vi "1. JKISM vs CSM.vi"() -> ()   [LabVIEW 2017]
uses:
  user.lib/_NEVSTOP/Communicable State Machine(CSM)/AdvanceAPI/CSM - Revert Arguments-Safe String.vi
  user.lib/_NEVSTOP/Communicable State Machine(CSM)/AdvanceAPI/CSM - Make String Arguments Safe.vi
  user.lib/_NEVSTOP/Communicable State Machine(CSM)/AdvanceAPI/CSM - Break Down Multiple States String.vi
  user.lib/_NEVSTOP/Communicable State Machine(CSM)/AdvanceAPI/CSM - Compact Multiple States.vi
  user.lib/_NEVSTOP/Communicable State Machine(CSM)/AdvanceAPI/CSM - Keywords.vi
  user.lib/_NEVSTOP/Communicable State Machine(CSM)/_Shared/Trim Single-line Text.vi
  user.lib/_NEVSTOP/Communicable State Machine(CSM)/Communicable State Machine.lvlib
panel:
  out "State History":string
  in  "Name (\"\" to Use UUID)":string="Event CSM"
  in  "Exit":bool
  # "Demonstrates the framework structures of the JKISM and CSM state machine templates. Both frameworks use string-based message queues to implement the core state machine."
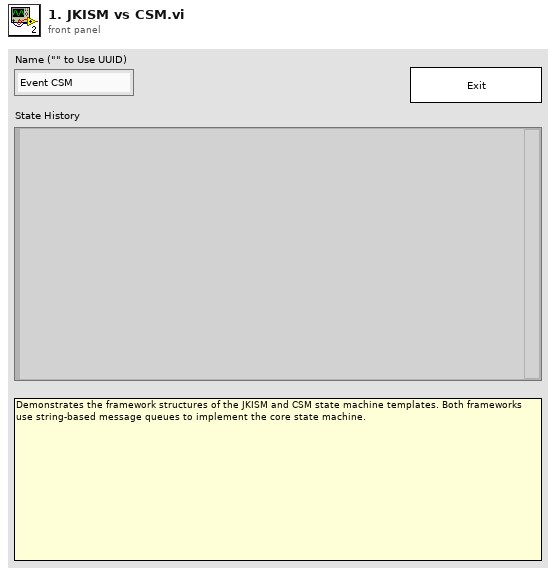
[diagram p1: front panel]
types:
  T1 = enum32{"Invalid", "Standard", "Closed", "Hidden", "Minimized", "Maximized"}
  T2 = enum32{"invalid app kind", "Development System", "Run Time System", "Student Edition", "Embedded LabVIEW", "Evaluation", "Custom"}
  T3 = cluster{"Core":cluster{"Current VI Reference":refnum<vi>, "Close Panel on Exit?":bool}, "Your Boolean data":bool, "Your string data":string}
  T4 = cluster{"Current VI Reference":refnum<vi>, "Close Panel on Exit?":bool}
  T5 = typedef "Communicable State Machine.lvlib/_CSM_Response Source Message.ctl" = cluster{"‘State":string, "’Arguments":string, "’Error":errorcluster}
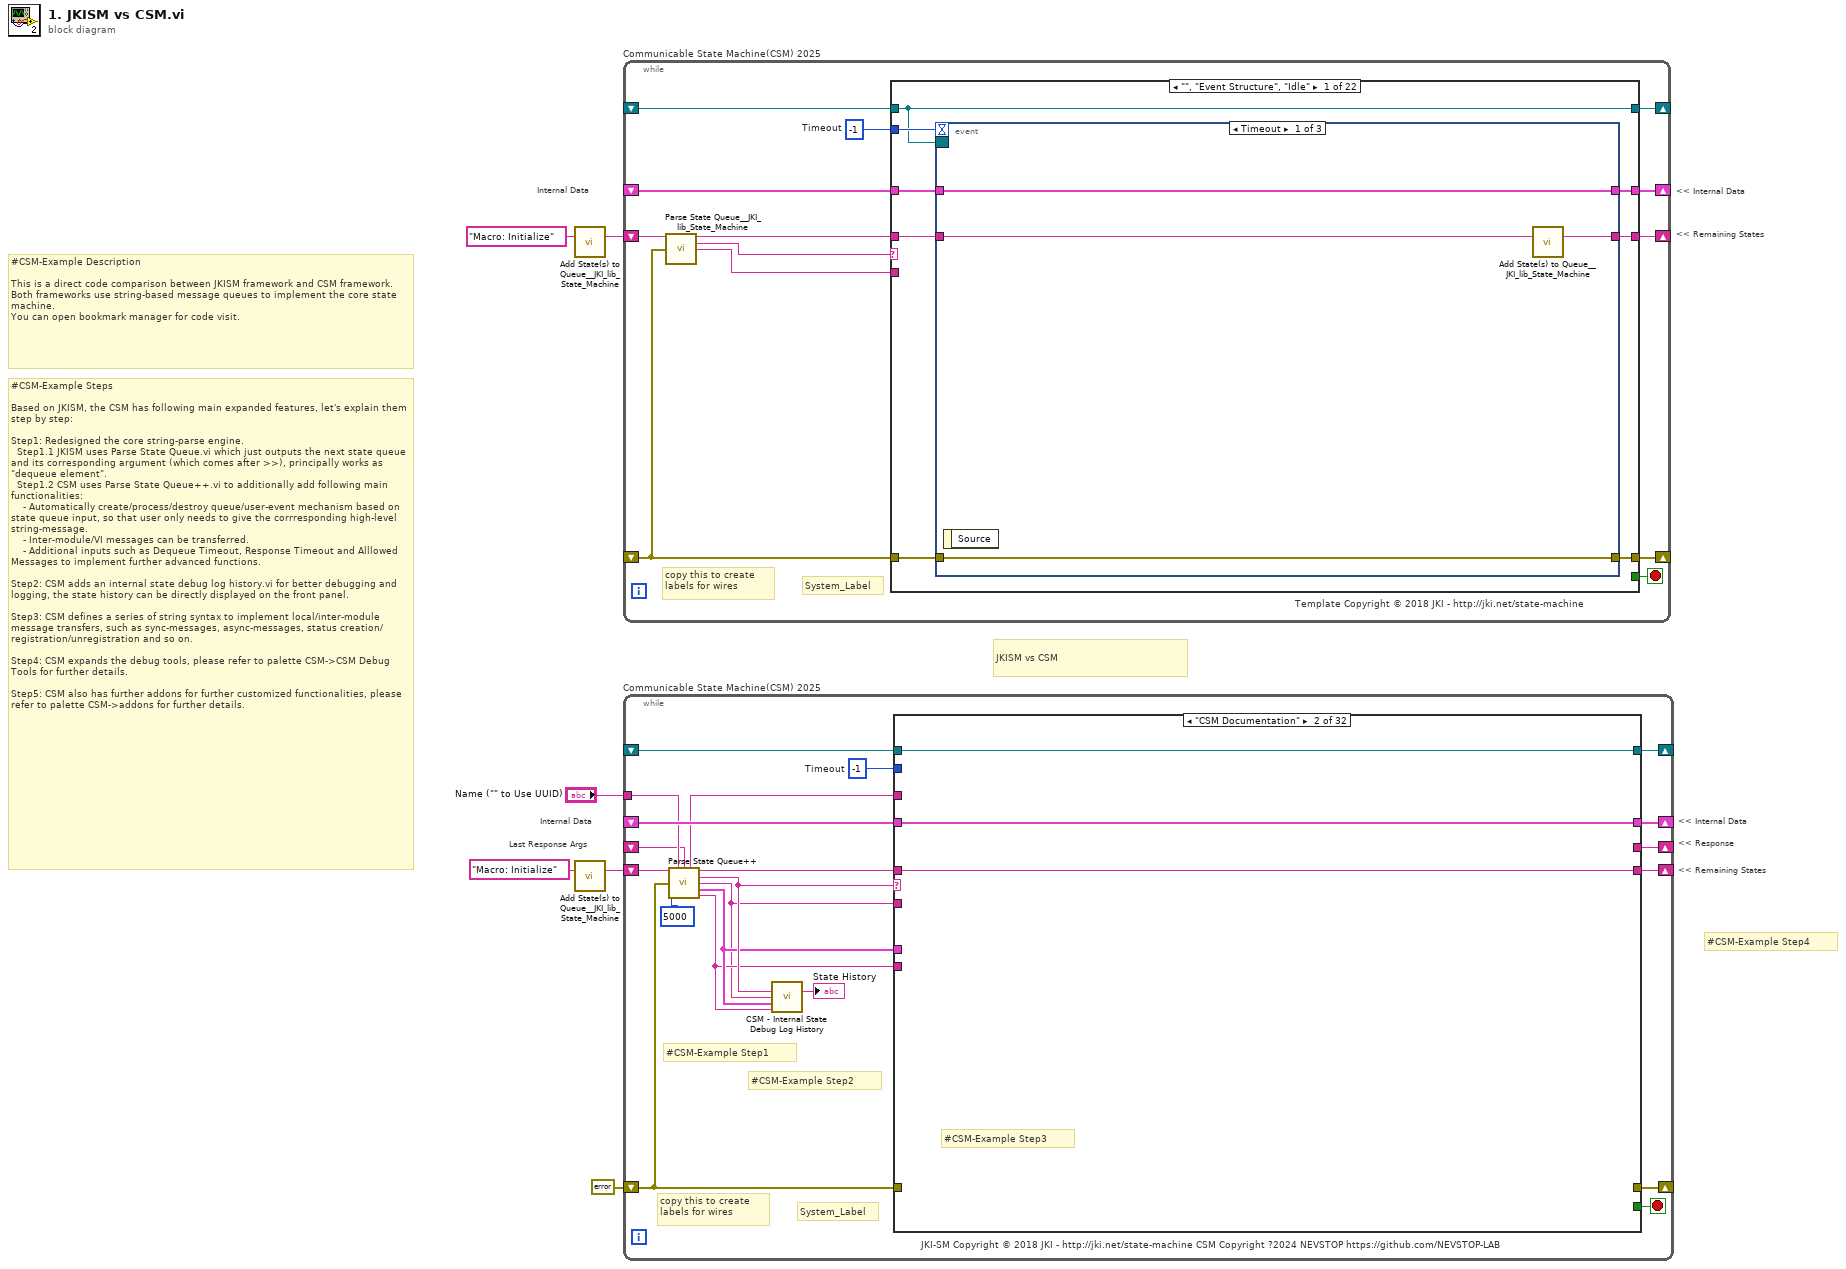
[diagram p0: block diagram]
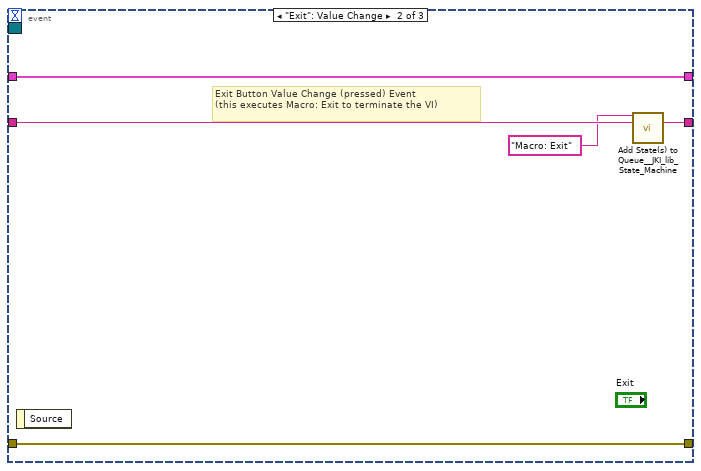
[diagram p2: hidden frame]
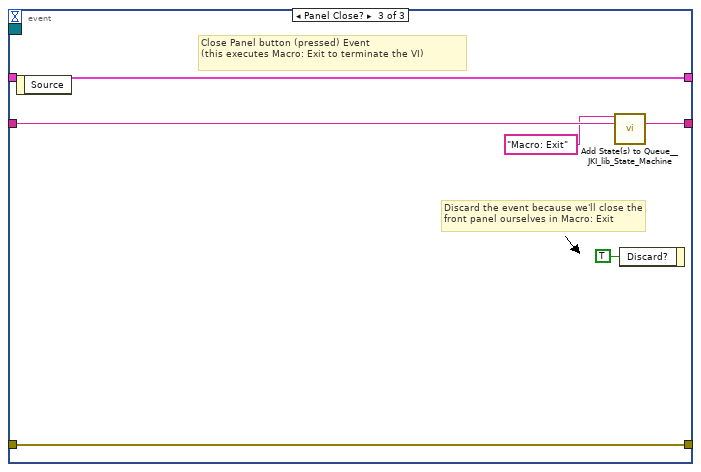
[diagram p3: hidden frame]
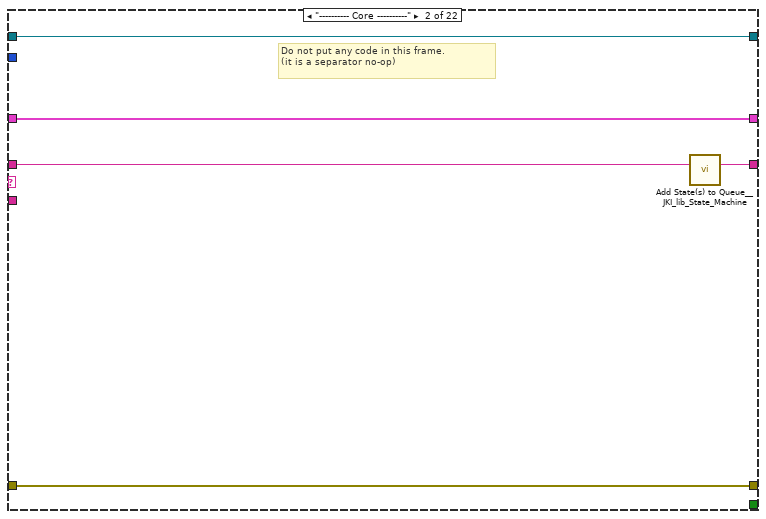
[diagram p4: hidden frame]
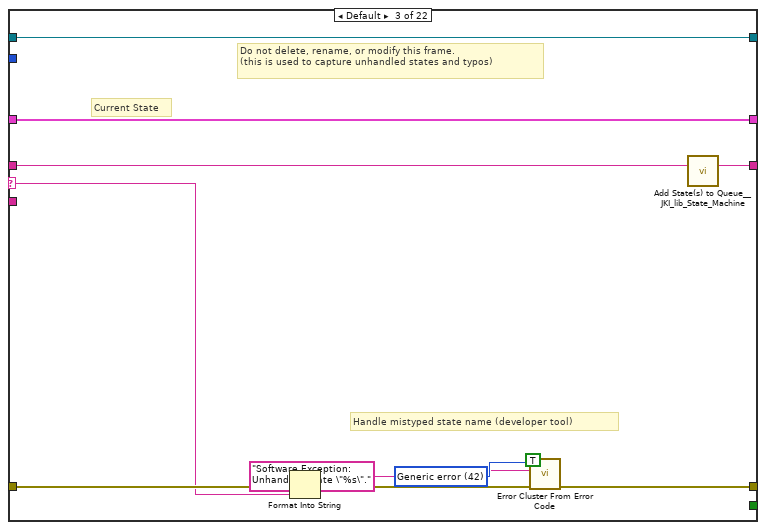
[diagram p5: hidden frame]
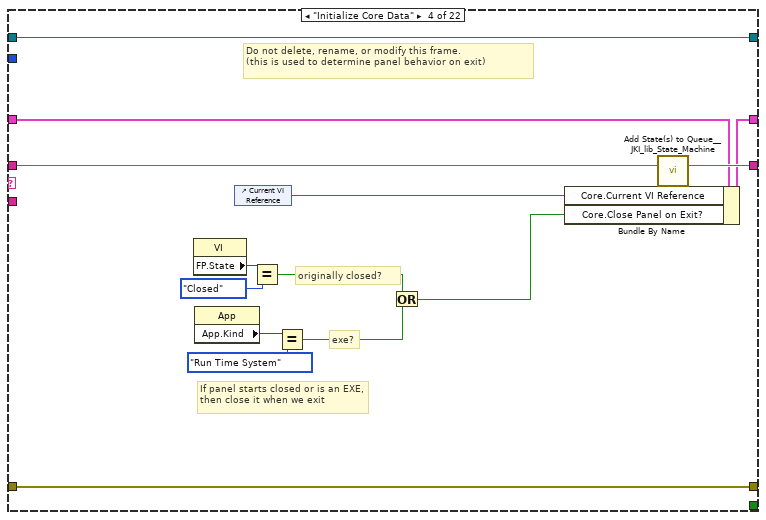
[diagram p6: hidden frame]
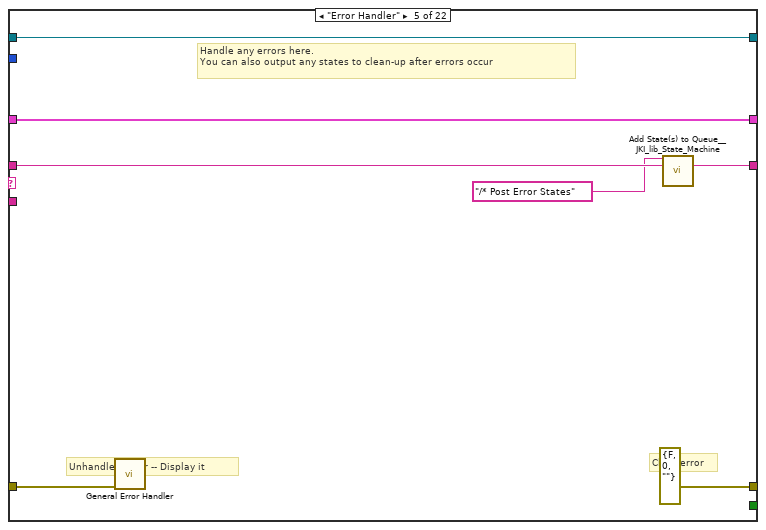
[diagram p7: hidden frame]
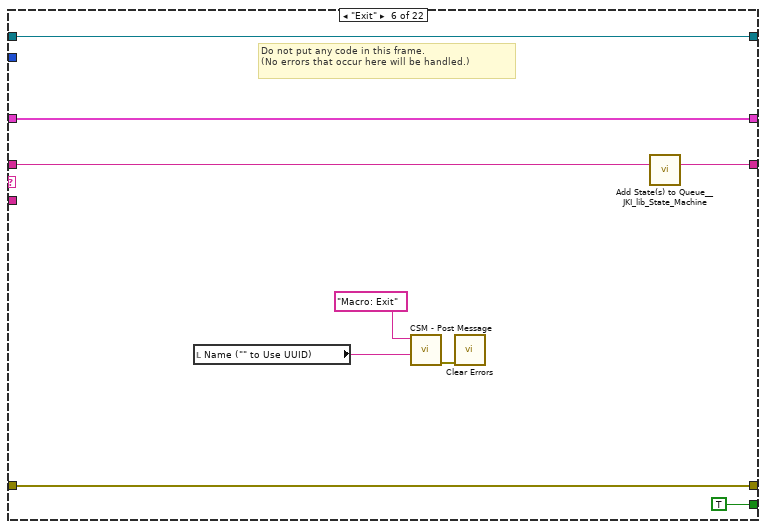
[diagram p8: hidden frame]
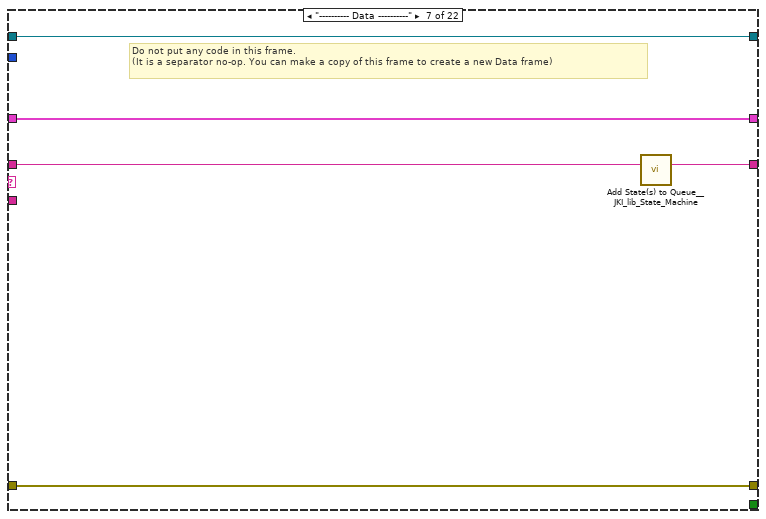
[diagram p9: hidden frame]
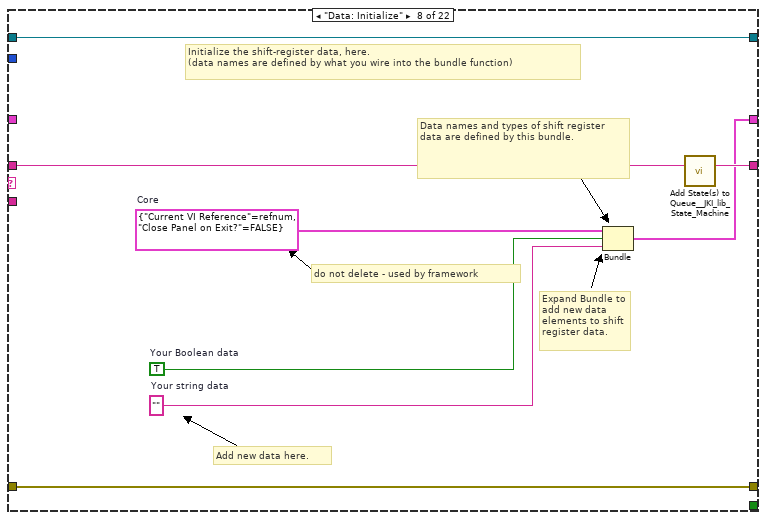
[diagram p10: hidden frame]
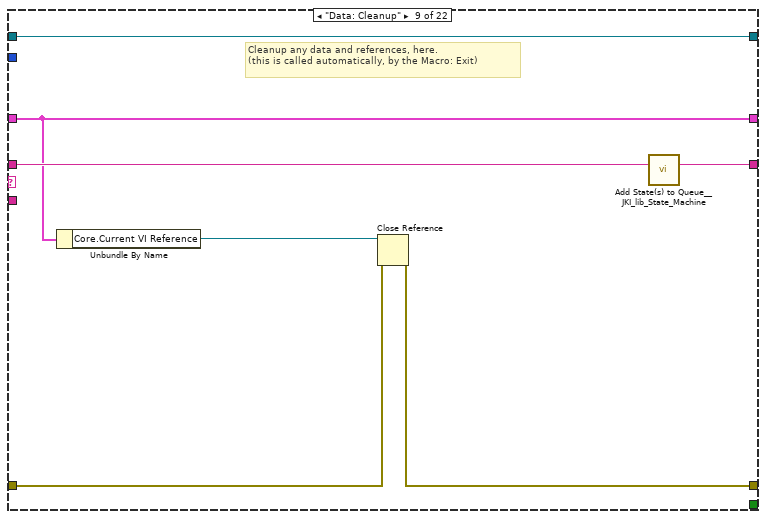
[diagram p11: hidden frame]
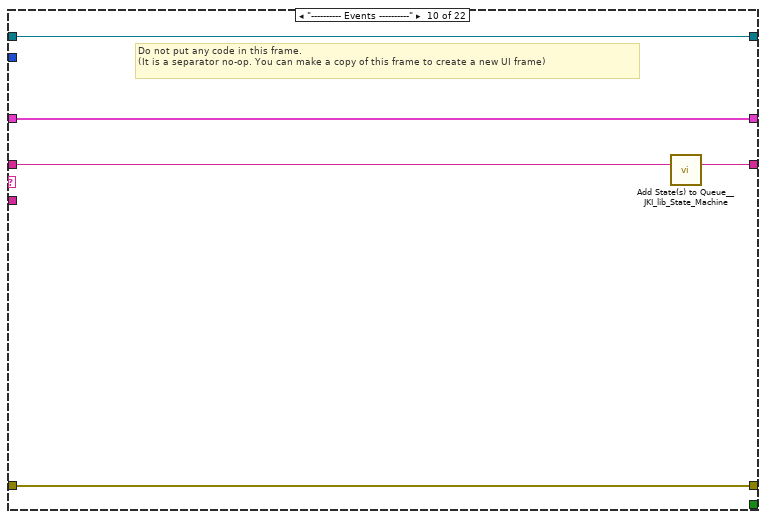
[diagram p12: hidden frame]
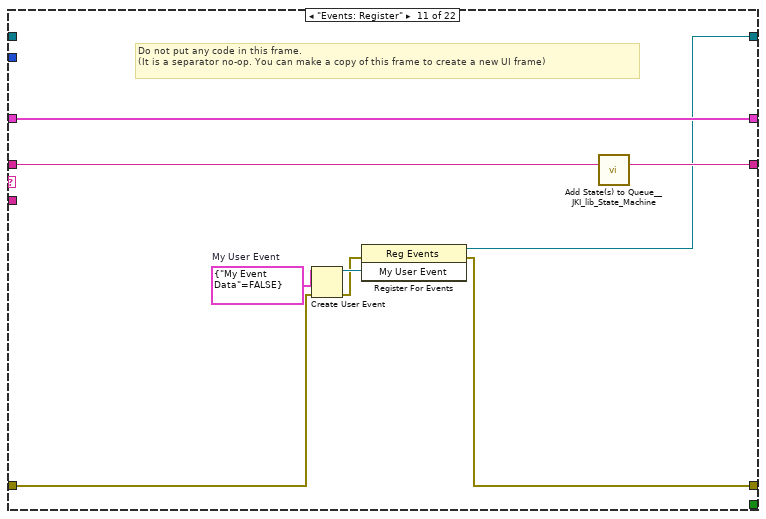
[diagram p13: hidden frame]
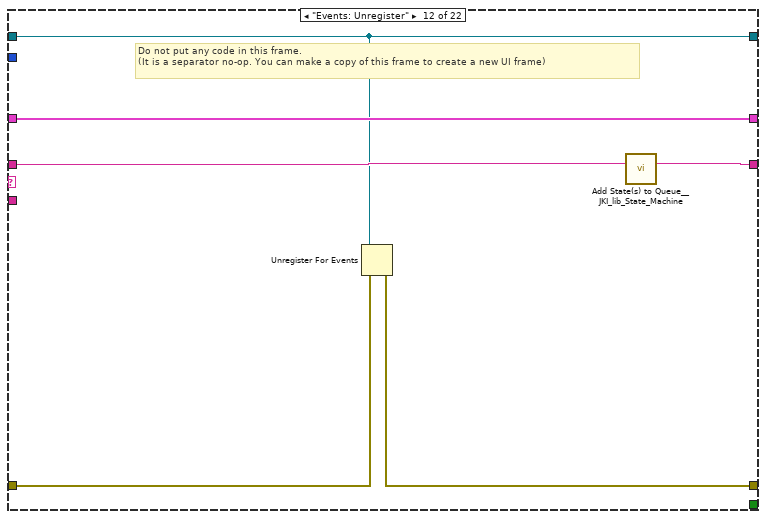
[diagram p14: hidden frame]
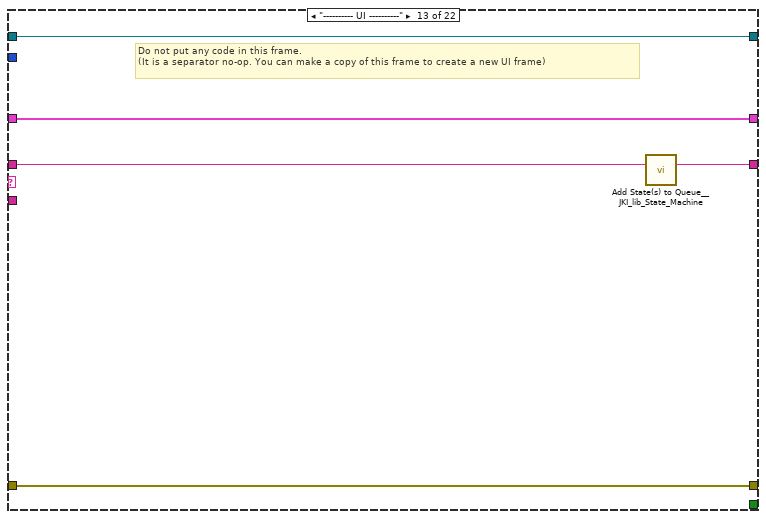
[diagram p15: hidden frame]
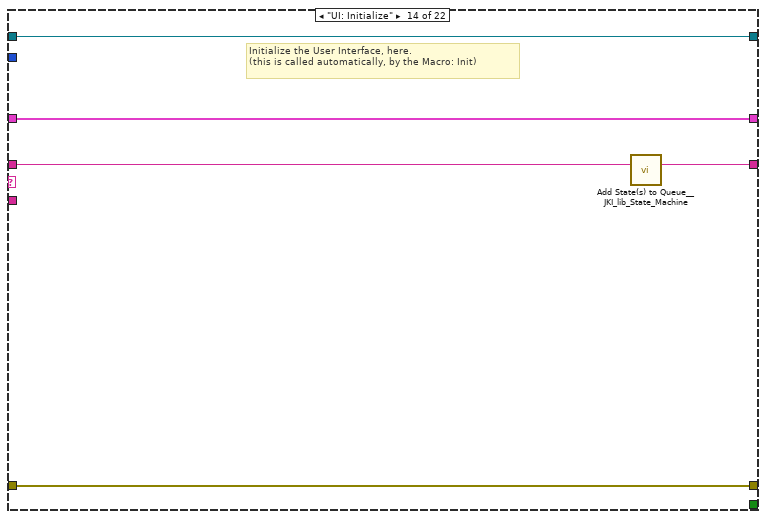
[diagram p16: hidden frame]
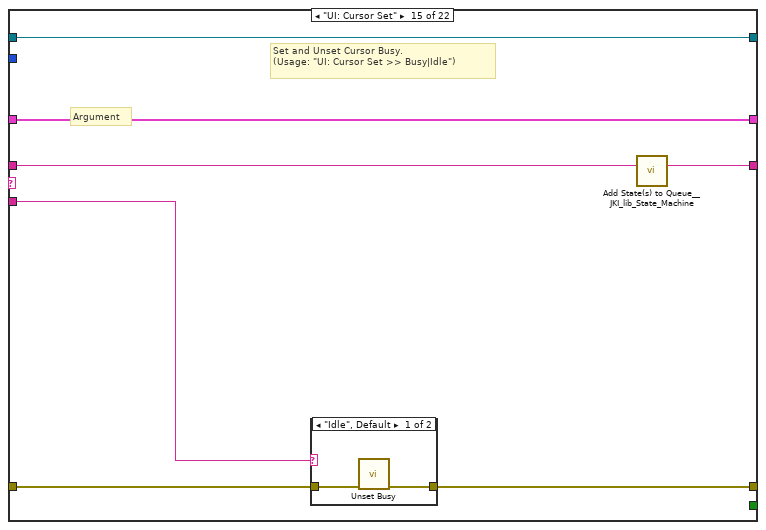
[diagram p17: hidden frame]
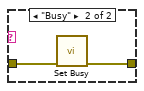
[diagram p18: hidden frame]
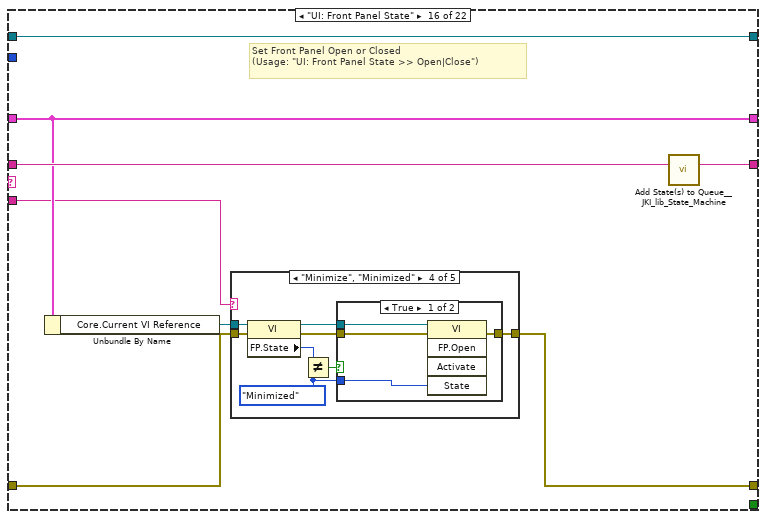
[diagram p19: hidden frame]
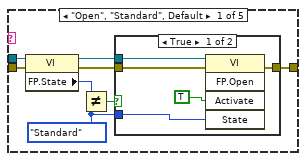
[diagram p20: hidden frame]
diagram:
  # "#CSM-Example Step4"
  # "#CSM-Example Steps\n\nBased on JKISM, the CSM has following main expanded features, let's explain them step by step:\n\nStep1: Redesigned the core string-parse engine.\n  Step1.1 JKISM uses Parse State Queue.vi which just outputs the next state queue and its corresponding argument (which comes after >>), principally works as \"dequeue element\".\n  Step1.2 CSM uses Parse State Queue++.vi to additionally add following main functionalities:\n    - Automatically create/process/destroy queue/user-event mechanism based on state queue input, so that user only needs to give the corrresponding high-level string-message.\n    - Inter-module/VI messages can be transferred.\n    - Additional inputs such as Dequeue Timeout, Response Timeout and Alllowed Messages to implement further advanced functions. \n\nStep2: CSM adds an internal state debug log history.vi for better debugging and logging, the state history can be directly displayed on the front panel.\n\nStep3: CSM defines a series of string syntax to implement local/inter-module message transfers, such as sync-messages, async-messages, status creation/registration/unregistration and so on.\n\nStep4: CSM expands the debug tools, please refer to palette CSM->CSM Debug Tools for further details.\n\nStep5: CSM also has further addons for further customized functionalities, please refer to palette CSM->addons for further details."
  # "#CSM-Example Description\n\nThis is a direct code comparison between JKISM framework and CSM framework. Both frameworks use string-based message queues to implement the core state machine.\nYou can open bookmark manager for code visit."
  # "JKISM vs CSM"
  # "<< Internal Data"
  # "<< Remaining States"
  # "Internal Data"
  # "Last Response Args"
  # "Internal Data"
  # "<< Internal Data"
  # "<< Response"
  # "<< Remaining States"
  n1 = call <vilib>:"Add State(s) to Queue__JKI_lib_State_Machine.vi"("State(s) in (\"\")"="Macro: Initialize") -> ("States Out"=w6:string)  [unwired: 14 in]
  n2 = call <vilib>:"Add State(s) to Queue__JKI_lib_State_Machine.vi"("State(s) in (\"\")"="Macro: Initialize" ("Init State(\"Macro: Initialize\")")) -> ("States Out"=w1:string)  [unwired: 14 in]
  n3 = while "Communicable State Machine(CSM) 2025" {
    shift-right: [w12] -> _
    shift-left: _ -> [w11]
    shift-right: [w15] -> _
    shift-left: _ -> [w9]
    shift-right: [w14] -> _
    shift-left: w6 -> [w16]
    shift-right: [w8] -> _
    shift-left: _ -> [w7]
    stop <- w13 stop-if-true
    w10 = -1  # Timeout
    # "copy this to create labels for wires"
    # "System_Label"
    # "Template Copyright © 2018 JKI - http://jki.net/state-machine"
    n4 = call <vilib>:"Parse State Queue__JKI_lib_State_Machine.vi"("State Queue"=w16, "Error In (no error)"=w9) -> ("Remaining States"=w18:string, "Current State"=w19:string, "Arguments"=w17:string)  [unwired: 11 in]
    n5 = case shown="\"\", \"Event Structure\", \"Idle\"" w19 {
      selector: w19 -> [_ _ w49 _ _ _ _ _ _ _ _ _ _ _ _ _ _ _ _ _ _ _]
      tunnel: w18 -> [w27 w47 w53 w73 w80 w89 w94 w102 w109 w114 w123 w129 w134 w139 w146 w158 w228 w234 w245 w250 w255 w260]
      tunnel: w17 -> [_ _ _ _ _ _ _ _ _ _ _ _ _ _ w141 w152 _ _ _ _ _ _]
      tunnel: w11 -> [w25 w44 w51 w66 w77 w87 w91 _ w104 w111 w121 w127 w131 w137 w144 w154 w225 w231 w242 w247 w252 w257]
      tunnel: [w24 w45 w55 w70 errorcluster {"status"=FALSE, "code"=0, "source"=""} ("error out") w86 w92 w99 w105 w112 w115 w124 w132 w136 w142 w155 w226 w232 w243 w248 w253 w258] -> w15
      tunnel: w9 -> [w23 w45 w54 w70 w76 w86 w92 w99 w106 w112 w117 w125 w132 w136 w143 w156 w226 w232 w243 w248 w253 w258]
      tunnel: [w26 w46 w52 w72 w79 w88 w93 w101 w108 w113 w122 w128 w133 w138 w145 w157 w227 w233 w244 w249 w254 w259] -> w14
      tunnel: [_ _ _ _ _ TRUE _ _ _ _ _ _ _ _ _ _ _ _ _ _ _ _] -> w13
      tunnel: [w22 w44 w51 w71 w77 w87 w91 w100 w104 w111 w121 w127 w131 w137 w144 w154 w225 w231 w242 w247 w252 w257] -> w12
      tunnel: w10 -> [w21 _ _ _ _ _ _ _ _ _ _ _ _ _ _ _ _ _ _ _ _ _]
      tunnel: [w20 w43 w48 w60 w74 w84 w90 w95 w103 w110 w118 w126 w130 w135 w140 w151 w224 w229 w235 w246 w251 w256] -> w8
      tunnel: w7 -> [w20 w43 w48 w60 w74 w84 w90 w95 w103 w110 _ w126 w130 w135 w140 w151 w224 w229 w235 w246 w251 w256]
      frame "", "Event Structure", "Idle" {
        n6 = event shown="[0] Timeout" {
          selector: w20 -> [_ _ _]
          dyn-events: _ -> [_ _ _]
          timeout: w21 -> [_ _ _]
          tunnel: w27 -> [w31 w36 w42]
          tunnel: [w30 w35 w41] -> w26
          tunnel: w25 -> [w28 w33 w39]
          tunnel: [w29 w34 w40] -> w24
          tunnel: w23 -> [w29 w34 w40]
          tunnel: [w28 w33 w39] -> w22
          event Timeout {
            n7 = event-data() -> ()  [unwired: 1 in, 1 out]
            n8 = call <vilib>:"Add State(s) to Queue__JKI_lib_State_Machine.vi"("State(s) in (\"\")"=w31) -> ("States Out"=w30:string)  [unwired: 14 in]
          }
          event "Exit": Value Change {
            # "Exit Button Value Change (pressed) Event\n(this executes Macro: Exit to terminate the VI)"
            n9 = event-data() -> ()  [unwired: 1 in, 1 out]
            n10 = call <vilib>:"Add State(s) to Queue__JKI_lib_State_Machine.vi"("State(s) in Front (\"\")"="Macro: Exit", "State(s) in (\"\")"=w36) -> ("States Out"=w35:string)  [unwired: 13 in]
          }
          event Panel Close? {
            # "Discard the event because we'll close the front panel ourselves in Macro: Exit"
            # "Close Panel button (pressed) Event\n(this executes Macro: Exit to terminate the VI)"
            n11 = event-data() -> ()  [unwired: 1 in, 1 out]
            n12 = call <vilib>:"Add State(s) to Queue__JKI_lib_State_Machine.vi"("State(s) in Front (\"\")"="Macro: Exit", "State(s) in (\"\")"=w42) -> ("States Out"=w41:string)  [unwired: 13 in]
            n13 = event-data("Discard?"=TRUE) -> ()  [unwired: 1 in, 1 out]
          }
        }
      }
      frame "---------- Core ----------" {
        # "Do not put any code in this frame.\n(it is a separator no-op)"
        n14 = call <vilib>:"Add State(s) to Queue__JKI_lib_State_Machine.vi"("State(s) in (\"\")"=w47) -> ("States Out"=w46:string)  [unwired: 14 in]
      }
      frame Default {
        w58 = 42 items=["No error", "Argument error", "Memory is full", "Out of zone", "End of file", "File already open", "Generic file I/O error", "File not found", "File permission error", "Disk is full", "Duplicate path", "Too many files open", "System feature not enabled", "Resource file not found", "Cannot add resource", "Resource not found", "Image not found", "Image memory error", "Pen does not exist", "Config type invalid", "Config token not found", "Config parse error", "Config memory error", "Bad external code format", "Bad external code offset", "External code not present", "Null window", "Destroy window error", "Null menu", "Print aborted", "Bad print record", "Print driver error", "Windows error during printing", "Memory error during printing", "Print dialog error", "Generic print error", "Invalid device refnum", "Device not found", "Device parameter error", "Device unit error", "Cannot open device", "Device call aborted", "Generic error", "Cancelled by user", "Object ID too low", "Object ID too high", "Object not in heap", "Unknown heap", "Unknown object (invalid DefProc)", "Unknown object (DefProc not in table)", "Message out of range", "Invalid (null) method", "Unknown message", "Manager call not supported", "Bad address", "Network operation in progress", "Network operation timed out", "Connection is busy", "Network attribute not supported", "Network error", "Address in use", "System out of memory", "Connection aborted", "Connection refused", "Not connected", "Already connected", "Connection closed", "Initialization error (interapplication manager)", "Bad occurrence", "Wait on unbound occurrence handler", "Occurrence queue overflow", "Datalog type conflict", "Unused", "Unrecognized type (interapplication manager)", "Memory corrupt", "Failed to make temporary DLL", "Old CIN version", "Drag socket not found", "Failed to load drop-object", "Failed to register OLE object", "Failed to release OLE object", "Format specifier type mismatch", "Unknown format specifier", "Too few format specifiers", "Too many format specifiers", "Scan failed", "Newer CIN version", "Error converting to variant", "Runtime menu error", "Password tampered", "Variant attribute not found", "Incompatible variant data type", "Event data is not available", "Event Store is not present", "Occurrence is not found", "Event Queue is not created", "Event info is not available", "Refnum passed is NULL", "Error retrieving Class GUID", "Error retrieving CoClass GUID", "Error retrieving TypeLib GUID.", "Bad built application magic bytes.", "Specific driver is different from the specific driver associated with the Logical Name.", "There is no session opened to the class driver.", "Max Error", "MAX - Error with config objects", "MAX - Error loading configuration", "MAX - Group not supported"]
        # "Current State"
        # "Do not delete, rename, or modify this frame.\n(this is used to capture unhandled states and typos)"
        # "Handle mistyped state name (developer tool)"
        n15 = Format Into String(format string="Software Exception: Unhandled State \"%s\"." ("message"), error in=w54, w49) -> (resulting string=w57:string, error out=w56:errorcluster)  [unwired: 1 in]
        n16 = call <vilib>:"Error Cluster From Error Code.vi"("show call chain? (False)"=TRUE, "error in (no error)"=w56, "error message (\"\")"=w57, "error code (0)"=w58) -> ("error out"=w55:errorcluster)  [unwired: 5 in]
        n17 = call <vilib>:"Add State(s) to Queue__JKI_lib_State_Machine.vi"("State(s) in (\"\")"=w53) -> ("States Out"=w52:string)  [unwired: 14 in]
      }
      frame "Initialize Core Data" {
        # "Do not delete, rename, or modify this frame.\n(this is used to determine panel behavior on exit)"
        # "originally closed?"
        # "exe?"
        # "If panel starts closed or is an EXE, then close it when we exit"
        n18 = property class="VI"() -> ("FP.State"=w63:T1)  [unwired: 2 in, 2 out]
        n19 = property class="App"() -> ("App.Kind"=w69:T2)  [unwired: 2 in, 2 out]
        n20 = control-ref of="Current VI Reference"() -> (w64:refnum<vi>)
        n21 = Equal?(x=w63, y=T1."Closed" ("Front Panel Window:State")) -> (x = y?=w61:bool)
        n22 = Equal?(x=w69, y=T2."Run Time System" ("Application:Kind")) -> (x = y?=w67:bool)
        n23 = Or(x=w61, y=w67) -> (x .or. y?=w65:bool)
        n24 = Bundle By Name(cluster=w66, "Core.Current VI Reference"=w64, "Core.Close Panel on Exit?"=w65) -> (w71:T3)
        n25 = call <vilib>:"Add State(s) to Queue__JKI_lib_State_Machine.vi"("State(s) in (\"\")"=w73) -> ("States Out"=w72:string)  [unwired: 14 in]
      }
      frame "Error Handler" {
        # "Unhandled Error -- Display it"
        # "Handle any errors here.\nYou can also output any states to clean-up after errors occur"
        # "Clear error"
        n26 = call <vilib>:"General Error Handler.vi"("error in (no error)"=w76) -> ()  [unwired: 10 in, 5 out]
        n27 = call <vilib>:"Add State(s) to Queue__JKI_lib_State_Machine.vi"("State(s) in Front (\"\")"="/* Post Error States", "State(s) in (\"\")"=w80) -> ("States Out"=w79:string)  [unwired: 13 in]
      }
      frame "Exit" {
        # "Do not put any code in this frame.\n(No errors that occur here will be handled.)"
        n28 = local read "Name (\"\" to Use UUID)"() -> (w83:string)
        n29 = call "CSM - Post Message.vi"("Target Module"=w83, "State"="Macro: Exit") -> ("error out"=w81:errorcluster)  [unwired: 9 in]
        n30 = call <vilib>:"Clear Errors.vi"("error in (no error)"=w81) -> ()  [unwired: 5 in, 2 out]
        n31 = call <vilib>:"Add State(s) to Queue__JKI_lib_State_Machine.vi"("State(s) in (\"\")"=w89) -> ("States Out"=w88:string)  [unwired: 14 in]
      }
      frame "---------- Data ----------" {
        # "Do not put any code in this frame.\n(It is a separator no-op. You can make a copy of this frame to create a new Data frame)"
        n32 = call <vilib>:"Add State(s) to Queue__JKI_lib_State_Machine.vi"("State(s) in (\"\")"=w94) -> ("States Out"=w93:string)  [unwired: 14 in]
      }
      frame "Data: Initialize" {
        w96 = T4 {"Current VI Reference"=refnum, "Close Panel on Exit?"=FALSE}  # Core
        w98 = TRUE  # Your Boolean data
        w97 = ""  # Your string data
        # "do not delete - used by framework"
        # "Expand Bundle to add new data elements to shift register data."
        # "Add new data here."
        # "Data names and types of shift register data are defined by this bundle."
        # "Initialize the shift-register data, here.\n(data names are defined by what you wire into the bundle function)"
        n33 = Bundle("Core"=w96, "Your Boolean data"=w98, "Your string data"=w97) -> (w100:T3)  [unwired: 1 in]
        n34 = call <vilib>:"Add State(s) to Queue__JKI_lib_State_Machine.vi"("State(s) in (\"\")"=w102) -> ("States Out"=w101:string)  [unwired: 14 in]
      }
      frame "Data: Cleanup" {
        # "Cleanup any data and references, here.\n(this is called automatically, by the Macro: Exit)"
        n35 = Unbundle By Name(w104) -> ("Core.Current VI Reference"=w107:refnum<vi>)
        n36 = Close Reference(reference=w107, error in (no error)=w106) -> (error out=w105:errorcluster)
        n37 = call <vilib>:"Add State(s) to Queue__JKI_lib_State_Machine.vi"("State(s) in (\"\")"=w109) -> ("States Out"=w108:string)  [unwired: 14 in]
      }
      frame "---------- Events ----------" {
        # "Do not put any code in this frame.\n(It is a separator no-op. You can make a copy of this frame to create a new UI frame)"
        n38 = call <vilib>:"Add State(s) to Queue__JKI_lib_State_Machine.vi"("State(s) in (\"\")"=w114) -> ("States Out"=w113:string)  [unwired: 14 in]
      }
      frame "Events: Register" {
        w119 = cluster{"My Event Data":bool} {"My Event Data"=FALSE}  # My User Event
        # "Do not put any code in this frame.\n(It is a separator no-op. You can make a copy of this frame to create a new UI frame)"
        n39 = Create User Event(user event datatype=w119, error in=w117) -> (user event=w120:refnum<user-event>, error out=w116:errorcluster)
        n40 = register-events(error in=w116, w120) -> (reference out=w118:refnum<event-registration>, error out=w115:errorcluster)  [unwired: 1 in]
        n41 = call <vilib>:"Add State(s) to Queue__JKI_lib_State_Machine.vi"("State(s) in (\"\")"=w123) -> ("States Out"=w122:string)  [unwired: 14 in]
      }
      frame "Events: Unregister" {
        # "Do not put any code in this frame.\n(It is a separator no-op. You can make a copy of this frame to create a new UI frame)"
        n42 = Unregister For Events(event registration refnum=w126, error in=w125) -> (error out=w124:errorcluster)
        n43 = call <vilib>:"Add State(s) to Queue__JKI_lib_State_Machine.vi"("State(s) in (\"\")"=w129) -> ("States Out"=w128:string)  [unwired: 14 in]
      }
      frame "---------- UI ----------" {
        # "Do not put any code in this frame.\n(It is a separator no-op. You can make a copy of this frame to create a new UI frame)"
        n44 = call <vilib>:"Add State(s) to Queue__JKI_lib_State_Machine.vi"("State(s) in (\"\")"=w134) -> ("States Out"=w133:string)  [unwired: 14 in]
      }
      frame "UI: Initialize" {
        # "Initialize the User Interface, here.\n(this is called automatically, by the Macro: Init)"
        n45 = call <vilib>:"Add State(s) to Queue__JKI_lib_State_Machine.vi"("State(s) in (\"\")"=w139) -> ("States Out"=w138:string)  [unwired: 14 in]
      }
      frame "UI: Cursor Set" {
        # "Argument"
        # "Set and Unset Cursor Busy.\n(Usage: \"UI: Cursor Set >> Busy|Idle\")"
        n46 = case shown="\"Idle\", Default" w141 {
          tunnel: w143 -> [w148 w150]
          tunnel: [w147 w149] -> w142
          frame "Idle", Default {
            n47 = call <vilib>:"Unset Busy.vi"("error in (no error)"=w148) -> ("error out"=w147:errorcluster)  [unwired: 10 in]
          }
          frame "Busy" {
            n48 = call <vilib>:"Set Busy.vi"("error in (no error)"=w150) -> ("error out"=w149:errorcluster)  [unwired: 9 in, 1 out]
          }
        }
        n49 = call <vilib>:"Add State(s) to Queue__JKI_lib_State_Machine.vi"("State(s) in (\"\")"=w146) -> ("States Out"=w145:string)  [unwired: 14 in]
      }
      frame "UI: Front Panel State" {
        # "Set Front Panel Open or Closed\n(Usage: \"UI: Front Panel State >> Open|Close\")"
        n50 = Unbundle By Name(w154) -> ("Core.Current VI Reference"=w153:refnum<vi>)
        n51 = case shown="\"Minimize\", \"Minimized\"" w152 {
          tunnel: w156 -> [w164 w179 w190 w203 w216]
          tunnel: [w166 w180 w192 w205 w218] -> w155
          tunnel: w153 -> [w165 w177 w191 w204 w217]
          frame "Open", "Standard", Default {
            w159 = T1."Standard" ("State")
            n52 = property class="VI"(reference=w165, error in=w164) -> (reference out=w162:refnum<vi>, error out=w163:errorcluster, "FP.State"=w161:T1)
            n53 = Not Equal?(x=w161, y=w159) -> (x != y?=w160:bool)
            n54 = case shown="True" w160 {
              tunnel: [w170 w172] -> w166
              tunnel: w163 -> [w169 w172]
              tunnel: w162 -> [w168 _]
              tunnel: w159 -> [w167 _]
              frame True {
                n55 = invoke class="VI" method="FP.Open"(reference=w168, error in=w169, "Activate"=TRUE, "State"=w167) -> (error out=w170:errorcluster)  [unwired: 1 in, 4 out]
              }
              frame False {
              }
            }
          }
          frame "Close", "Closed" {
            n56 = property class="VI"(reference=w177, error in=w179) -> (reference out=w176:refnum<vi>, error out=w178:errorcluster, "FP.State"=w174:T1)
            n57 = Not Equal?(x=w174, y=T1."Closed" ("Front Panel Window:State")) -> (x != y?=w173:bool)
            n58 = case shown="True" w173 {
              tunnel: [w181 w184] -> w180
              tunnel: w178 -> [w181 w183]
              tunnel: w176 -> [_ w182]
              frame False {
              }
              frame True {
                n59 = invoke class="VI" method="FP.Close"(reference=w182, error in=w183) -> (error out=w184:errorcluster)  [unwired: 1 in, 2 out]
              }
            }
          }
          frame "Hidden", "Hide" {
            w185 = T1."Hidden" ("State")
            n60 = property class="VI"(reference=w191, error in=w190) -> (reference out=w188:refnum<vi>, error out=w189:errorcluster, "FP.State"=w187:T1)
            n61 = Not Equal?(x=w187, y=w185) -> (x != y?=w186:bool)
            n62 = case shown="True" w186 {
              tunnel: [w196 w197] -> w192
              tunnel: w189 -> [w195 w197]
              tunnel: w188 -> [w194 _]
              tunnel: w185 -> [w193 _]
              frame True {
                n63 = invoke class="VI" method="FP.Open"(reference=w194, error in=w195, "State"=w193) -> (error out=w196:errorcluster)  [unwired: 2 in, 4 out]
              }
              frame False {
              }
            }
          }
          frame "Minimize", "Minimized" {
            w198 = T1."Minimized" ("State")
            n64 = property class="VI"(reference=w204, error in=w203) -> (reference out=w201:refnum<vi>, error out=w202:errorcluster, "FP.State"=w200:T1)
            n65 = Not Equal?(x=w200, y=w198) -> (x != y?=w199:bool)
            n66 = case shown="True" w199 {
              tunnel: [w209 w210] -> w205
              tunnel: w202 -> [w208 w210]
              tunnel: w201 -> [w207 _]
              tunnel: w198 -> [w206 _]
              frame True {
                n67 = invoke class="VI" method="FP.Open"(reference=w207, error in=w208, "State"=w206) -> (error out=w209:errorcluster)  [unwired: 2 in, 4 out]
              }
              frame False {
              }
            }
          }
          frame "Maximize", "Maximized" {
            w211 = T1."Maximized" ("State")
            n68 = property class="VI"(reference=w217, error in=w216) -> (reference out=w214:refnum<vi>, error out=w215:errorcluster, "FP.State"=w213:T1)
            n69 = Not Equal?(x=w213, y=w211) -> (x != y?=w212:bool)
            n70 = case shown="True" w212 {
              tunnel: [w222 w223] -> w218
              tunnel: w215 -> [w221 w223]
              tunnel: w214 -> [w220 _]
              tunnel: w211 -> [w219 _]
              frame True {
                n71 = invoke class="VI" method="FP.Open"(reference=w220, error in=w221, "State"=w219) -> (error out=w222:errorcluster)  [unwired: 2 in, 4 out]
              }
              frame False {
              }
            }
          }
        }
        n72 = call <vilib>:"Add State(s) to Queue__JKI_lib_State_Machine.vi"("State(s) in (\"\")"=w158) -> ("States Out"=w157:string)  [unwired: 14 in]
      }
      frame "---------- Macro ----------" {
        # "Do not put any code in this frame.\n(It is a separator no-op. You can make a copy of this frame to create a new Macro frame)"
        n73 = call <vilib>:"Add State(s) to Queue__JKI_lib_State_Machine.vi"("State(s) in (\"\")"=w228) -> ("States Out"=w227:string)  [unwired: 14 in]
      }
      frame "Macro: Initialize" {
        # "Initialization Macro\n(This is called once, when the VI starts)"
        n74 = call <vilib>:"Add State(s) to Queue__JKI_lib_State_Machine.vi"("State(s) in Front (\"\")"="Data: Initialize\nInitialize Core Data\nEvents: Register\nUI: Initialize\nUI: Front Panel State >> Open", "State(s) in (\"\")"=w234) -> ("States Out"=w233:string)  [unwired: 13 in]
      }
      frame "Macro: Exit" {
        # "Exit Macro\n(This is called once, when the VI exits)"
        n75 = Unbundle By Name(w242) -> ("Core.Close Panel on Exit?"=w241:bool)
        n76 = Select(t="UI: Front Panel State >> Close", s=w241, f="") -> (s? t:f=w238:string)
        n77 = call <vilib>:"Add State(s) to Queue__JKI_lib_State_Machine.vi"("State(s) in (\"\")"=w238, "State(s) at Back (\"\")"="Data: Cleanup\nEvents: Unregister\nExit") -> ("States Out"=w236:string)  [unwired: 13 in]
        n78 = call <vilib>:"Add State(s) to Queue__JKI_lib_State_Machine.vi"("State(s) in Front (\"\")"=w236, "State(s) in (\"\")"=w245) -> ("States Out"=w244:string)  [unwired: 13 in]
      }
      frame "---------- New Category ----------" {
        # "Template Separator\n(You can make a copy of, or modify, this frame)"
        n79 = call <vilib>:"Add State(s) to Queue__JKI_lib_State_Machine.vi"("State(s) in (\"\")"=w250) -> ("States Out"=w249:string)  [unwired: 14 in]
      }
      frame "New Category: 1" {
        # "Your code here.\n(You can make a copy of, or modify, this frame)"
        n80 = call <vilib>:"Add State(s) to Queue__JKI_lib_State_Machine.vi"("State(s) in (\"\")"=w255) -> ("States Out"=w254:string)  [unwired: 14 in]
      }
      frame "New Category: 2" {
        # "Your code here.\n(You can make a copy of, or modify, this frame)"
        n81 = call <vilib>:"Add State(s) to Queue__JKI_lib_State_Machine.vi"("State(s) in (\"\")"=w260) -> ("States Out"=w259:string)  [unwired: 14 in]
      }
    }
  }
  n82 = while "Communicable State Machine(CSM) 2025" {
    shift-right: [w276] -> _
    shift-left: _ -> [w275]
    shift-right: [w279] -> _
    shift-left: errorcluster {"status"=FALSE, "code"=0, "source"=""} ("error out") -> [w273]
    shift-right: [w278] -> _
    shift-left: w1 -> [w280]
    tunnel: "Name (\"\" to Use UUID)" -> [w268]
    shift-right: [w271] -> _
    shift-left: _ -> [w263]
    shift-right: [w270] -> _
    shift-left: _ -> [w269]
    stop <- w277 stop-if-true
    w274 = -1  # Timeout
    # "#CSM-Example Step2"
    # "#CSM-Example Step1"
    # "copy this to create labels for wires"
    # "System_Label"
    # "JKI-SM Copyright © 2018 JKI - http://jki.net/state-machine CSM Copyright ?2024 NEVSTOP https://github.com/NEVSTOP-LAB"
    n83 = call "Parse State Queue++.vi"("State Queue"=w280, "Name (\"\" to Use UUID)"=w268, "Response Arguments"=w263, "Previous Error"=w273, "Response Timeout (-2 Use Global Settings)"=5000 ("Response Timeout(1000ms)")) -> ("Name Used"=w264:string, "Remaining States"=w281:string, "Current State"=w267:string, "Arguments"=w262:string, ">> Response Source Message >>"=w266:T5, ">> Source CSM >>"=w265:string)  [unwired: 5 in]
    n84 = call "CSM - Internal State Debug Log History.vi"("State"=w267, "Arguments (\"\")"=w262, ">> Response Source Message >>"=w266, "Source (\"\")"=w265) -> ("Debug Log"=→"State History":string)  [unwired: 11 in]
    n85 = case shown="\"CSM Documentation\"" w267 {
      selector: w267 -> [_ _ _ w312 _ _ _ _ _ _ _ _ _ _ _ _ _ _ _ _ _ _ _ _ _ _ _ _ _ _ _ _]
      tunnel: w281 -> [w283 w304 w309 w318 w324 w330 w356 w364 w371 w381 w390 w403 w408 w412 w419 w425 w429 w436 w440 w444 w448 w454 w465 w529 w534 w545 w548 w552 w555 w559 w563 w567]
      tunnel: w262 -> [_ _ _ _ _ w328 w352 w359 w367 w375 _ _ _ _ _ _ _ _ _ _ _ w450 w460 _ _ _ _ _ _ _ _ _]
      tunnel: w275 -> [w289 w303 w306 w316 w323 w336 w357 w362 w369 w379 w389 w397 w406 w410 _ w421 w427 w435 w439 w442 w446 w452 w462 w527 w532 w543 w547 w551 w554 w557 w561 w565]
      tunnel: [w288 _ w307 w310 w325 errorcluster {"status"=FALSE, "code"=0, "source"=""} ("error out") w349 w358 w365 w378 _ _ _ _ _ w422 _ w430 w438 _ _ w451 w463 _ _ _ _ _ _ _ _ _] -> w279
      tunnel: w273 -> [w282 _ w307 w311 w325 w334 w350 w360 w366 _ _ _ _ _ _ _ _ _ _ _ _ _ _ _ _ _ _ _ _ _ _ _]
      tunnel: [w290 w304 w308 w317 w324 w332 w355 w363 w370 w382 w390 w402 w407 w411 w418 w424 w428 w436 w440 w443 w447 w453 w464 w528 w533 w544 w548 w552 w555 w558 w562 w566] -> w278
      tunnel: [_ _ _ _ _ _ TRUE _ _ _ _ _ TRUE _ _ _ _ _ _ _ _ _ _ _ _ _ _ _ _ _ _ _] -> w277
      tunnel: [w287 w303 w306 w316 w323 w336 w357 w362 w369 w380 w389 w401 w406 w410 w417 w421 w427 w435 w439 w442 w446 w452 w462 w527 w532 w543 w547 w551 w554 w557 w561 w565] -> w276
      tunnel: w274 -> [w285 _ _ _ _ _ _ _ _ _ _ _ _ _ _ _ _ _ _ _ _ _ _ _ _ _ _ _ _ _ _ _]
      tunnel: w265 -> [_ _ _ _ _ w327 _ _ _ w376 _ _ _ _ _ _ _ _ _ _ _ _ _ _ _ _ _ _ _ _ _ _]
      tunnel: w266 -> [_ _ _ _ _ w326 _ _ _ w377 _ _ _ _ _ _ _ _ _ _ _ _ _ _ _ _ _ _ _ _ _ _]
      tunnel: [_ _ _ "" w319 _ _ _ _ _ _ _ _ _ _ _ _ _ _ _ _ _ _ _ _ _ _ "API1 Response" _ _ _ _] -> w271
      tunnel: [w286 w302 w305 w314 w322 w335 w353 w361 w368 w383 w388 w391 w404 w409 w413 w420 w426 w434 w437 w441 w445 w449 w459 w526 w530 w536 w546 w550 w553 w556 w560 w564] -> w270
      tunnel: w269 -> [w286 w302 w305 w314 w322 w335 w353 w361 w368 w383 w388 w391 w404 w409 w413 w420 w426 _ w437 w441 w445 w449 w459 w526 w530 w536 w546 w550 w553 w556 w560 w564]
      tunnel: w264 -> [_ _ _ w313 _ _ w351 _ _ _ _ _ _ _ _ _ _ w433 _ _ _ _ _ _ _ _ _ _ _ _ _ _]
      frame "", "Event Structure", "Idle" {
        n86 = call "Timeout Selector.vi"("Remaining States"=w283, "Timeout Expected"=w285) -> ("Timeout"=w284:i32)  [unwired: 5 in]
        n87 = event shown="[0] Timeout" {
          selector: w286 -> [_ _ _]
          dyn-events: _ -> [_ _ _]
          timeout: w284 -> [_ _ _]
          tunnel: w283 -> [w294 w295 w301]
          tunnel: [w293 w295 w300] -> w290
          tunnel: w289 -> [w292 w296 w299]
          tunnel: [w291 _ _] -> w288
          tunnel: [w292 w296 w299] -> w287
          tunnel: w282 -> [w291 _ _]
          event Timeout {
            n88 = event-data() -> ()  [unwired: 1 in, 1 out]
            n89 = call <vilib>:"Add State(s) to Queue__JKI_lib_State_Machine.vi"("State(s) in (\"\")"=w294) -> ("States Out"=w293:string)  [unwired: 14 in]
          }
          event User Event {
            n90 = event-data() -> ()  [unwired: 1 in, 1 out]
          }
          event Panel Close? {
            n91 = event-data() -> ()  [unwired: 1 in, 1 out]
            n92 = call <vilib>:"Add State(s) to Queue__JKI_lib_State_Machine.vi"("State(s) in Front (\"\")"="Macro: Exit", "State(s) in (\"\")"=w301) -> ("States Out"=w300:string)  [unwired: 13 in]
            n93 = event-data("Discard?"=TRUE) -> ()  [unwired: 1 in, 1 out]
          }
        }
      }
      frame "CSM Documentation" {
        # "#CSM-Example Step3"
      }
      frame "---------- Core ----------" {
        n94 = call <vilib>:"Add State(s) to Queue__JKI_lib_State_Machine.vi"("State(s) in (\"\")"=w309) -> ("States Out"=w308:string)  [unwired: 14 in]
      }
      frame Default {
        n95 = call "CSM Unhandled State Error.vi"("error in (no error)"=w311, "Current State"=w312, "CSM Name"=w313) -> ("error out"=w310:errorcluster)  [unwired: 8 in]
        n96 = call <vilib>:"Add State(s) to Queue__JKI_lib_State_Machine.vi"("State(s) in (\"\")"=w318) -> ("States Out"=w317:string)  [unwired: 14 in]
      }
      frame "VI Reference" {
        n97 = Unbundle By Name(w323) -> ("Core"=w321:T4)
        n98 = Unbundle By Name(w321) -> ("Current VI Reference"=w320:refnum<vi>)
        n99 = call "CSM - Convert Data to HexStr.vi"("Variant"=w320) -> ("HEX String (0-9,A-F)"=w319:string)  [unwired: 8 in]
      }
      frame "Error Handler" {
        # "Clear error"
        n100 = case shown="Error" w334 {
          selector: w334 -> [_ w343]
          tunnel: [w341 w345] -> w331
          tunnel: w330 -> [w341 w344]
          tunnel: [w340 w343] -> w329
          tunnel: w328 -> [w342 _]
          tunnel: w327 -> [_ _]
          tunnel: w326 -> [_ _]
          frame No Error {
            n101 = call "CSM - Convert Argument to Error.vi"("Argument"=w342) -> ("Error"=w340:errorcluster)  [unwired: 4 in]
            n102 = flat-sequence {
              frame #0 {
              }
            }
          }
          frame Error {
            n103 = call "CSM - Convert Error to Argument.vi"("Error"=w343) -> ("Argument"=w347:string)  [unwired: 4 in]
            n104 = call <vilib>:"Build State String with Arguments__JKI_lib_State_Machine.vi"("Arguments (\"\")"=w347, "State"="Error Occurred" ("Status with Arguments")) -> ("State with Arguments"=w346:string)  [unwired: 4 in]
            n105 = call "CSM - Broadcast Status Change.vi"("Status With Arguments"=w346, "State Queue"=w344) -> ("Remaining States"=w345:string)  [unwired: 13 in]
          }
        }
        n106 = disable-structure shown="Enabled" {
          disable-tunnel: w329 -> [w338 w339]
          frame Enabled {
            # "Unhandled Error -- Display it"
            n107 = call <vilib>:"General Error Handler.vi"("error in (no error)"=w338) -> ()  [unwired: 10 in, 5 out]
          }
          frame Disabled {
            n108 = call <vilib>:"Clear Errors.vi"("error in (no error)"=w339) -> ()  [unwired: 5 in, 2 out]
          }
        }
        n109 = call <vilib>:"Add State(s) to Queue__JKI_lib_State_Machine.vi"("State(s) in Front (\"\")"="// Post Error States", "State(s) in (\"\")"=w331) -> ("States Out"=w332:string)  [unwired: 13 in]
      }
      frame "Critical Error" {
        n110 = call "CSM Critical Error.vi"("error in (no error)"=w350, "Arugments (As Reason)"=w352, "CSM Name"=w351) -> ("error out"=w349:errorcluster)  [unwired: 8 in]
        n111 = call <vilib>:"Add State(s) to Queue__JKI_lib_State_Machine.vi"("State(s) in (\"\")"=w356) -> ("States Out"=w355:string)  [unwired: 14 in]
      }
      frame "Target Timeout Error" {
        n112 = call "CSM Target Timeout Error.vi"("error in (no error)"=w360, "Arguments (As CSM Name)"=w359) -> ("error out"=w358:errorcluster)  [unwired: 9 in]
        n113 = call <vilib>:"Add State(s) to Queue__JKI_lib_State_Machine.vi"("State(s) in (\"\")"=w364) -> ("States Out"=w363:string)  [unwired: 14 in]
      }
      frame "Target Error" {
        n114 = call "CSM Target Error.vi"("error in (no error)"=w366, "Arguments (As CSM Name)"=w367) -> ("error out"=w365:errorcluster)  [unwired: 9 in]
        n115 = call <vilib>:"Add State(s) to Queue__JKI_lib_State_Machine.vi"("State(s) in (\"\")"=w371) -> ("States Out"=w370:string)  [unwired: 14 in]
      }
      frame "Async Response", "Response" {
        n116 = Unbundle(w377) -> ("‘State"=w374:string, "’Arguments"=w373:string, "’Error"=w372:errorcluster)
        n117 = case shown="Default" w374 {
          tunnel: [w384] -> w382
          tunnel: w381 -> [w385]
          tunnel: [w387] -> w380
          tunnel: w379 -> [w387]
          tunnel: [w386] -> w378
          tunnel: w372 -> [w386]
          tunnel: w376 -> [_]
          tunnel: w375 -> [_]
          tunnel: w373 -> [_]
          frame Default {
            n118 = call <vilib>:"Add State(s) to Queue__JKI_lib_State_Machine.vi"("State(s) in (\"\")"=w385) -> ("States Out"=w384:string)  [unwired: 14 in]
          }
        }
      }
      frame "Async Message Posted" {
      }
      frame "Initialize Core Data" {
        # "originally closed?"
        # "exe?"
        # "If panel starts closed or is an EXE, then close it when we exit"
        n119 = property class="VI"() -> ("FP.State"=w394:T1)  [unwired: 2 in, 2 out]
        n120 = property class="App"() -> ("App.Kind"=w400:T2)  [unwired: 2 in, 2 out]
        n121 = control-ref of="Current VI Reference"() -> (w395:refnum<vi>)
        n122 = Equal?(x=w394, y=T1."Closed" ("Front Panel Window:State")) -> (x = y?=w392:bool)
        n123 = Equal?(x=w400, y=T2."Run Time System" ("Application:Kind")) -> (x = y?=w398:bool)
        n124 = Or(x=w392, y=w398) -> (x .or. y?=w396:bool)
        n125 = Bundle By Name(cluster=w397, "Core.Current VI Reference"=w395, "Core.Close Panel on Exit?"=w396) -> (w401:T3)
        n126 = call <vilib>:"Add State(s) to Queue__JKI_lib_State_Machine.vi"("State(s) in (\"\")"=w403) -> ("States Out"=w402:string)  [unwired: 14 in]
      }
      frame "Exit" {
        n127 = call <vilib>:"Add State(s) to Queue__JKI_lib_State_Machine.vi"("State(s) in (\"\")"=w408) -> ("States Out"=w407:string)  [unwired: 14 in]
      }
      frame "---------- Data ----------" {
        n128 = call <vilib>:"Add State(s) to Queue__JKI_lib_State_Machine.vi"("State(s) in (\"\")"=w412) -> ("States Out"=w411:string)  [unwired: 14 in]
      }
      frame "Data: Initialize" {
        w414 = T4 {"Current VI Reference"=refnum, "Close Panel on Exit?"=FALSE}  # Core
        w416 = TRUE  # Your Boolean data
        w415 = ""  # Your string data
        n129 = Bundle("Core"=w414, "Your Boolean data"=w416, "Your string data"=w415) -> (w417:T3)  [unwired: 1 in]
        n130 = call <vilib>:"Add State(s) to Queue__JKI_lib_State_Machine.vi"("State(s) in (\"\")"=w419) -> ("States Out"=w418:string)  [unwired: 14 in]
      }
      frame "Data: Cleanup" {
        n131 = Unbundle By Name(w421) -> ("Core.Current VI Reference"=w423:refnum<vi>)
        n132 = Close Reference(reference=w423) -> (error out=w422:errorcluster)  [unwired: 1 in]
        n133 = call <vilib>:"Add State(s) to Queue__JKI_lib_State_Machine.vi"("State(s) in (\"\")"=w425) -> ("States Out"=w424:string)  [unwired: 14 in]
      }
      frame "---------- Events ----------" {
        n134 = call <vilib>:"Add State(s) to Queue__JKI_lib_State_Machine.vi"("State(s) in (\"\")"=w429) -> ("States Out"=w428:string)  [unwired: 14 in]
      }
      frame "Events: Register" {
        n135 = call "CSM - Get New State Notifier Event.vi"("Name (\"\" to Use UUID) In"=w433) -> ("error out"=w431:errorcluster, "New State Notifier Event"=w432:refnum<user-event>)  [unwired: 9 in]
        n136 = register-events(error in=w431, w432) -> (reference out=w434:refnum<event-registration>, error out=w430:errorcluster)  [unwired: 1 in]
      }
      frame "Events: Unregister" {
        n137 = Unregister For Events(event registration refnum=w437) -> (error out=w438:errorcluster)  [unwired: 1 in]
      }
      frame "---------- UI ----------" {
        n138 = call <vilib>:"Add State(s) to Queue__JKI_lib_State_Machine.vi"("State(s) in (\"\")"=w444) -> ("States Out"=w443:string)  [unwired: 14 in]
      }
      frame "UI: Initialize" {
        n139 = call <vilib>:"Add State(s) to Queue__JKI_lib_State_Machine.vi"("State(s) in (\"\")"=w448) -> ("States Out"=w447:string)  [unwired: 14 in]
      }
      frame "UI: Cursor Set" {
        # "Argument"
        n140 = disable-structure shown="Default" {
          disable-tunnel: [w456 _] -> w451
          disable-tunnel: w450 -> [w455 _]
          frame condition #0 (active) {
            n141 = case shown="\"Idle\", Default" w455 {
              tunnel: [w457 w458] -> w456
              frame "Idle", Default {
                n142 = call <vilib>:"Unset Busy.vi"() -> ("error out"=w457:errorcluster)  [unwired: 11 in]
              }
              frame "Busy" {
                n143 = call <vilib>:"Set Busy.vi"() -> ("error out"=w458:errorcluster)  [unwired: 10 in, 1 out]
              }
            }
          }
          frame condition #1 {
          }
        }
        n144 = call <vilib>:"Add State(s) to Queue__JKI_lib_State_Machine.vi"("State(s) in (\"\")"=w454) -> ("States Out"=w453:string)  [unwired: 14 in]
      }
      frame "UI: Front Panel State" {
        # "Argument"
        n145 = Unbundle By Name(w462) -> ("Core.Current VI Reference"=w461:refnum<vi>)
        n146 = case shown="\"Minimize\", \"Minimized\"" w460 {
          tunnel: [w472 w485 w496 w508 w520] -> w463
          tunnel: w461 -> [w471 w483 w495 w507 w519]
          frame "Open", "Standard", Default {
            w466 = T1."Standard" ("State")
            n147 = property class="VI"(reference=w471) -> (reference out=w469:refnum<vi>, error out=w470:errorcluster, "FP.State"=w468:T1)  [unwired: 1 in]
            n148 = Not Equal?(x=w468, y=w466) -> (x != y?=w467:bool)
            n149 = case shown="True" w467 {
              tunnel: [w476 w478] -> w472
              tunnel: w470 -> [w475 w478]
              tunnel: w469 -> [w474 _]
              tunnel: w466 -> [w473 _]
              frame True {
                n150 = invoke class="VI" method="FP.Open"(reference=w474, error in=w475, "Activate"=TRUE, "State"=w473) -> (error out=w476:errorcluster)  [unwired: 1 in, 4 out]
              }
              frame False {
              }
            }
          }
          frame "Close", "Closed" {
            n151 = property class="VI"(reference=w483) -> (reference out=w482:refnum<vi>, error out=w484:errorcluster, "FP.State"=w480:T1)  [unwired: 1 in]
            n152 = Not Equal?(x=w480, y=T1."Closed" ("Front Panel Window:State")) -> (x != y?=w479:bool)
            n153 = case shown="True" w479 {
              tunnel: [w486 w489] -> w485
              tunnel: w484 -> [w486 w488]
              tunnel: w482 -> [_ w487]
              frame False {
              }
              frame True {
                n154 = invoke class="VI" method="FP.Close"(reference=w487, error in=w488) -> (error out=w489:errorcluster)  [unwired: 1 in, 2 out]
              }
            }
          }
          frame "Hidden", "Hide" {
            w490 = T1."Hidden" ("State")
            n155 = property class="VI"(reference=w495) -> (reference out=w493:refnum<vi>, error out=w494:errorcluster, "FP.State"=w492:T1)  [unwired: 1 in]
            n156 = Not Equal?(x=w492, y=w490) -> (x != y?=w491:bool)
            n157 = case shown="True" w491 {
              tunnel: [w500 w501] -> w496
              tunnel: w494 -> [w499 w501]
              tunnel: w493 -> [w498 _]
              tunnel: w490 -> [w497 _]
              frame True {
                n158 = invoke class="VI" method="FP.Open"(reference=w498, error in=w499, "State"=w497) -> (error out=w500:errorcluster)  [unwired: 2 in, 4 out]
              }
              frame False {
              }
            }
          }
          frame "Minimize", "Minimized" {
            w502 = T1."Minimized" ("State")
            n159 = property class="VI"(reference=w507) -> (reference out=w505:refnum<vi>, error out=w506:errorcluster, "FP.State"=w504:T1)  [unwired: 1 in]
            n160 = Not Equal?(x=w504, y=w502) -> (x != y?=w503:bool)
            n161 = case shown="False" w503 {
              tunnel: [w512 w513] -> w508
              tunnel: w506 -> [w511 w513]
              tunnel: w505 -> [w510 _]
              tunnel: w502 -> [w509 _]
              frame True {
                n162 = invoke class="VI" method="FP.Open"(reference=w510, error in=w511, "State"=w509) -> (error out=w512:errorcluster)  [unwired: 2 in, 4 out]
              }
              frame False {
              }
            }
          }
          frame "Maximize", "Maximized" {
            w514 = T1."Maximized" ("State")
            n163 = property class="VI"(reference=w519) -> (reference out=w517:refnum<vi>, error out=w518:errorcluster, "FP.State"=w516:T1)  [unwired: 1 in]
            n164 = Not Equal?(x=w516, y=w514) -> (x != y?=w515:bool)
            n165 = case shown="True" w515 {
              tunnel: [w524 w525] -> w520
              tunnel: w518 -> [w523 w525]
              tunnel: w517 -> [w522 _]
              tunnel: w514 -> [w521 _]
              frame True {
                n166 = invoke class="VI" method="FP.Open"(reference=w522, error in=w523, "State"=w521) -> (error out=w524:errorcluster)  [unwired: 2 in, 4 out]
              }
              frame False {
              }
            }
          }
        }
        n167 = call <vilib>:"Add State(s) to Queue__JKI_lib_State_Machine.vi"("State(s) in (\"\")"=w465) -> ("States Out"=w464:string)  [unwired: 14 in]
      }
      frame "---------- Macro ----------" {
        n168 = call <vilib>:"Add State(s) to Queue__JKI_lib_State_Machine.vi"("State(s) in (\"\")"=w529) -> ("States Out"=w528:string)  [unwired: 14 in]
      }
      frame "Macro: Initialize" {
        w531 = "Data: Initialize\nInitialize Core Data\nEvents: Register\nUI: Initialize\nUI: Front Panel State >> Open"  # Data: Initialize Initialize Core Data Events: Register UI: Initialize UI: Front Panel State >> Open
        n169 = call <vilib>:"Add State(s) to Queue__JKI_lib_State_Machine.vi"("State(s) in Front (\"\")"=w531, "State(s) in (\"\")"=w534) -> ("States Out"=w533:string)  [unwired: 13 in]
      }
      frame "Macro: Exit" {
        n170 = Unbundle By Name(w543) -> ("Core.Close Panel on Exit?"=w542:bool)
        n171 = Select(t="UI: Front Panel State >> Close", s=w542, f="") -> (s? t:f=w539:string)
        n172 = call <vilib>:"Add State(s) to Queue__JKI_lib_State_Machine.vi"("State(s) in Front (\"\")"="//Exit Sub-Modules ", "State(s) in (\"\")"=w539, "State(s) at Back (\"\")"="Data: Cleanup\nEvents: Unregister\nExit") -> ("States Out"=w537:string)  [unwired: 12 in]
        n173 = call <vilib>:"Add State(s) to Queue__JKI_lib_State_Machine.vi"("State(s) in Front (\"\")"=w537, "State(s) in (\"\")"=w545) -> ("States Out"=w544:string)  [unwired: 13 in]
      }
      frame "---------- API ----------" {
      }
      frame "API: API1" {
      }
      frame "API: API2" {
      }
      frame "---------- Action ----------" {
        n174 = call <vilib>:"Add State(s) to Queue__JKI_lib_State_Machine.vi"("State(s) in (\"\")"=w559) -> ("States Out"=w558:string)  [unwired: 14 in]
      }
      frame "Action: action1" {
        n175 = call <vilib>:"Add State(s) to Queue__JKI_lib_State_Machine.vi"("State(s) in (\"\")"=w563) -> ("States Out"=w562:string)  [unwired: 14 in]
      }
      frame "Action: action2" {
        n176 = call <vilib>:"Add State(s) to Queue__JKI_lib_State_Machine.vi"("State(s) in (\"\")"=w567) -> ("States Out"=w566:string)  [unwired: 14 in]
      }
    }
  }
